vi "select data.vi"() -> ()   [LabVIEW 2020]
uses:
  source/Database OOP/Database Libraries/ADODB/ADODB Class/ADODB.lvclass
  source/Database OOP/Database Libraries/ADODB/UDL Connection Class/UDL Connection.lvclass
  C:/Users/User/Desktop/Raman Program/LV-Database-OOP/source/Database OOP/Database Libraries/Database Interfaces/Database Connection Class/Database Connection.lvclass
panel:
  out "Data":string[][](table)
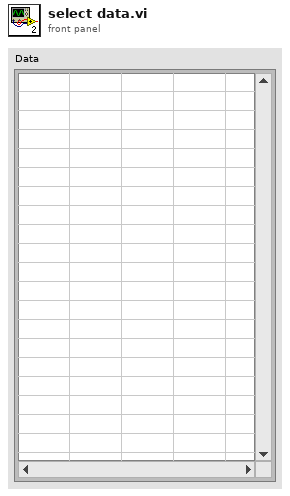
[diagram p1: front panel]
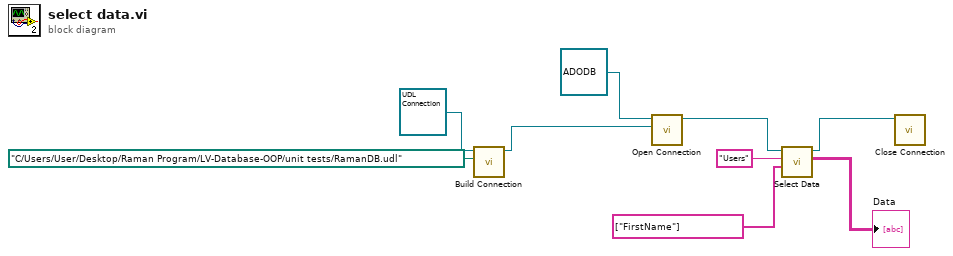
[diagram p0: block diagram]
diagram:
  n1 = call "Build Connection.vi"("*.udl file path"=path "C:/Users/User/Desktop/Raman Program/LV-Database-OOP/unit tests/RamanDB.udl", "UDL Connection in"=refnum<class "UDL Connection.lvclass"> refnum) -> ("UDL Connection out"=w2:refnum<class "UDL Connection.lvclass">)  [unwired: 8 in, 1 out]
  n2 = call-dynamic "Open Connection.vi"("Connection"=w2, "ADODB in"=refnum<class "ADODB.lvclass"> refnum) -> ("ADODB out"=w7:refnum<class "ADODB.lvclass">)  [unwired: 8 in, 1 out]
  n3 = call-dynamic "Select Data.vi"("Columns"=string[] ["FirstName"], "Table"="Users", "ADODB in"=w7) -> ("Data"=→"Data":string[][], "ADODB out"=w6:refnum<class "ADODB.lvclass">)  [unwired: 6 in, 1 out]
  n4 = call-dynamic "Close Connection.vi"("ODBC in"=w6) -> ()  [unwired: 9 in, 2 out]
